vi "Fct_Preparation_Data_Enregistrement.vi"(4 "Motif":string, 5 "Temperature":i32, 6 "Humidité":string, 7 "Vitesse vent":i32, 9 "Direction Vent":string, 10 "Luminosité":i32, 11 "Précipitation":i32) -> (3 "Chaîne":string)   [LabVIEW 2017]
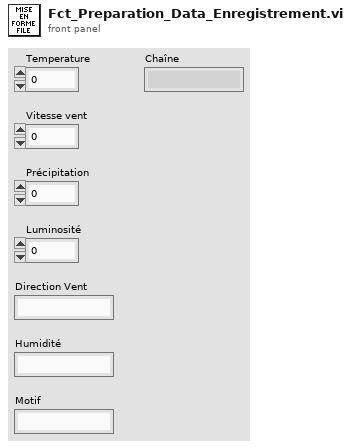
[diagram p1: front panel]
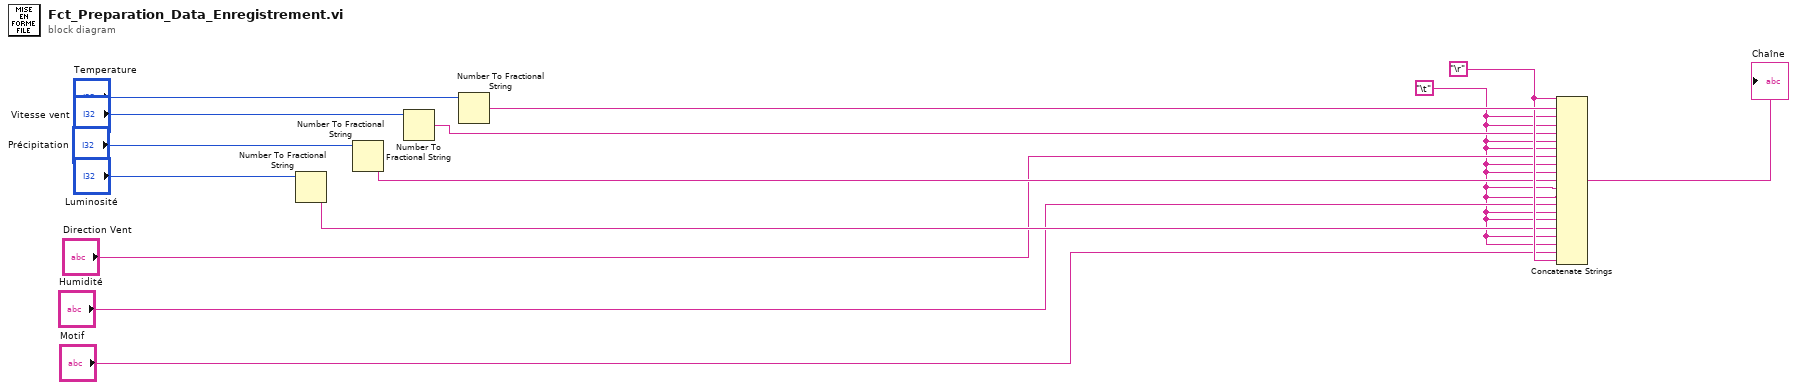
[diagram p0: block diagram]
diagram:
  w1 = "\t"
  w8 = "\r"
  n1 = Number To Fractional String(number="Luminosité") -> (F-format string=w7:string)  [unwired: 3 in]
  n2 = Number To Fractional String(number="Précipitation") -> (F-format string=w4:string)  [unwired: 3 in]
  n3 = Number To Fractional String(number="Vitesse vent") -> (F-format string=w2:string)  [unwired: 3 in]
  n4 = Number To Fractional String(number="Temperature") -> (F-format string=w10:string)  [unwired: 3 in]
  n5 = Concatenate Strings(w8, w10, w1, w1, w2, w1, w1, "Direction Vent", w1, w1, w4, w1, w1, "Humidité", w1, w1, w7, w1, w1, "Motif", w8) -> (→"Chaîne":string)
